vi "Configure Mediator.vi"(8 "Framework Instance Alias":string, 9 "Event Log Instance":refnum<class "LoggerReference.lvclass">, 10 "MediatorBusMonitor Type":refnum<class "IMediatorBusMonitor.lvclass">, 11 "Mediator in":refnum<class "IMediator.lvclass">) -> (3 "Mediator out":refnum<class "IMediator.lvclass">)   [LabVIEW 2017, in "IMediator.lvlib" / "IMediator.lvclass"]
uses:
  IMediator.lvclass
  IMediatorBusMonitor/IMediatorBusMonitor.lvclass
  gpm_packages/@cs/event-logger/Source/Composed Log/LoggerReference/LoggerReference.lvclass
  IMediator.lvclass/IMediator.ctl
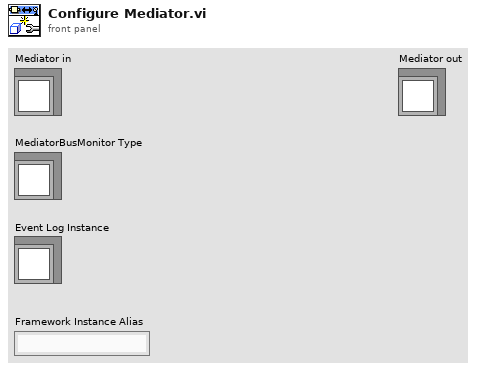
[diagram p1: front panel]
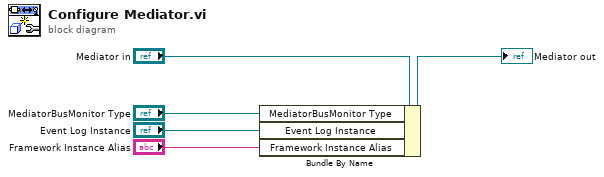
[diagram p0: block diagram]
diagram:
  n1 = Bundle By Name(cluster="Mediator in", "MediatorBusMonitor Type"="MediatorBusMonitor Type", "Event Log Instance"="Event Log Instance", "Framework Instance Alias"="Framework Instance Alias") -> (→"Mediator out":refnum<class "IMediator.lvclass">)
